vi "SMA.vi"(0 "System no.":i32=1 min=1 max=4 step=1, 2 "Pad axes":string[](array[string]), 3 "Stage axes":string[](array[string]), 5 "error in":errorcluster) -> (19 "error out":errorcluster)   [LabVIEW 2020]
doc: "Enables control of the specified axes with the (optional) manual control pad. Pad axes are axis IDs of the manual control pad (for 1 pad A-F, for 2 pads A-L). Stage axes are the corresponding axis IDs of connected stages to be controlled."
panel:
  # "Enables control of the specified axes with the (optional) \nmanual control pad. Pad axes are axis IDs of the manual\ncontrol pad (for 1 pad A-F, for 2 pads A-L), Stage axes are\nthe corresponding axis IDs of connected stages to be controlled."
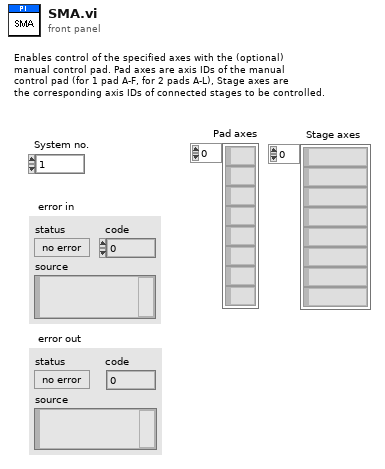
[diagram p1: front panel]
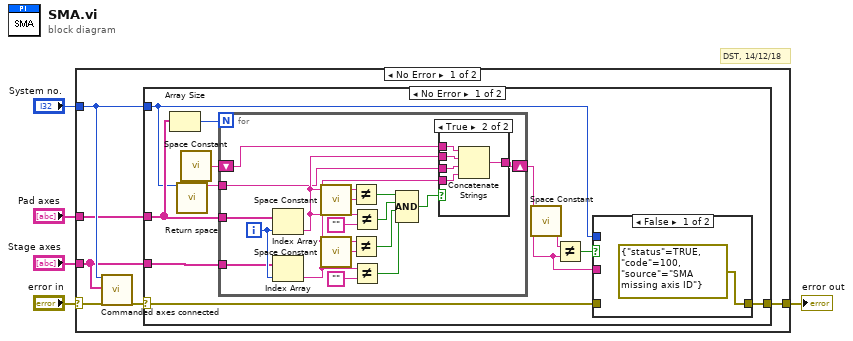
[diagram p0: block diagram]
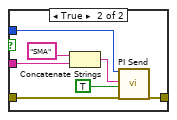
[diagram p2: hidden frame]
diagram:
  # "DST, 14/12/18"
  n1 = case shown="No Error" "error in" {
    selector: "error in" -> [w7 w55]
    tunnel: [w11 w55] -> w5
    tunnel: "System no." -> [w10 _]
    tunnel: "Pad axes" -> [w9 _]
    tunnel: "Stage axes" -> [w8 _]
    frame No Error {
      n2 = call "Commanded axes connected.vi"("System no."=w10, "Commanded axes"=w8, "error in"=w7) -> ("error out"=w6:errorcluster)  [unwired: 16 out]
      n3 = case shown="No Error" w6 {
        selector: w6 -> [w12 w54]
        tunnel: w9 -> [w22 _]
        tunnel: [w17 w54] -> w11
        tunnel: w8 -> [w19 _]
        tunnel: w10 -> [w13 _]
        frame No Error {
          n4 = Array Size(array=w22) -> (size(s)=w15:i32)
          n5 = call "Return space.vi"("System no."=w13) -> ("String out"=w14:string)  [unwired: 1 in, 17 out]
          n6 = call <vilib>:"Space Constant.vi"() -> ("String"=w21:string)
          n7 = for {
            N: w15 -> [_]
            tunnel: w22 -> [w36]
            shift-right: [w45] -> w18
            shift-left: w21 -> [w46]
            tunnel: w19 -> [w34]
            tunnel: w14 -> [w31]
            i -> [w35]
            n8 = Index Array(array=w36, index=w35) -> (element=w44:string)
            n9 = Index Array(array=w34, index=w35) -> (element=w33:string)
            n10 = call <vilib>:"Space Constant.vi"() -> ("String"=w47:string)
            n11 = call <vilib>:"Space Constant.vi"() -> ("String"=w42:string)
            n12 = Not Equal?(x=w44, y=w47) -> (x != y?=w40:bool)
            n13 = Not Equal?(x=w33, y=w42) -> (x != y?=w38:bool)
            n14 = Not Equal?(x=w44, y="") -> (x != y?=w39:bool)
            n15 = Not Equal?(x=w33, y="") -> (x != y?=w37:bool)
            n16 = Compound Arithmetic op=AND(w40, w39, w38, w37) -> (w32:bool)
            n17 = case shown="True" w32 {
              tunnel: w46 -> [w48 w53]
              tunnel: w44 -> [_ w51]
              tunnel: [w48 w52] -> w45
              tunnel: w33 -> [_ w50]
              tunnel: w31 -> [_ w49]
              frame False {
              }
              frame True {
                n18 = Concatenate Strings(w53, w51, w49, w50) -> (w52:string)
              }
            }
          }
          n19 = call <vilib>:"Space Constant.vi"() -> ("String"=w20:string)
          n20 = Not Equal?(x=w20, y=w18) -> (x != y?=w16:bool)
          n21 = case shown="False" w16 {
            tunnel: w18 -> [_ w28]
            tunnel: w12 -> [_ w26]
            tunnel: w13 -> [_ w25]
            tunnel: [errorcluster {"status"=TRUE, "code"=100, "source"="SMA missing axis ID"} ("error out") w24] -> w17
            frame False {
            }
            frame True {
              n22 = Concatenate Strings("SMA", w28) -> (w27:string)
              n23 = call "PI Send.vi"("System no."=w25, "String to send"=w27, "Attach termination char.?"=TRUE ("Attach Linefeed?"), "error in"=w26) -> ("error out"=w24:errorcluster)  [unwired: 2 in, 13 out]
            }
          }
        }
        frame Error {
        }
      }
    }
    frame Error {
    }
  }
  "error out" <- w5
